vi "步骤循环执行.vi"(0 "通知器输出":refnum<notifier>, 1 "停止":bool, 3 "error in (no error)":errorcluster caption="错误输入（无错误）") -> (7 "组合框":string(combo)="暂停", 10 "error out":errorcluster caption="错误输出")   [LabVIEW 2016]
panel:
  out "报警器":i32
  out "电磁阀2":i32
  out "电磁阀1":i32
  out "蠕动泵":i32
  out "气泵":i32
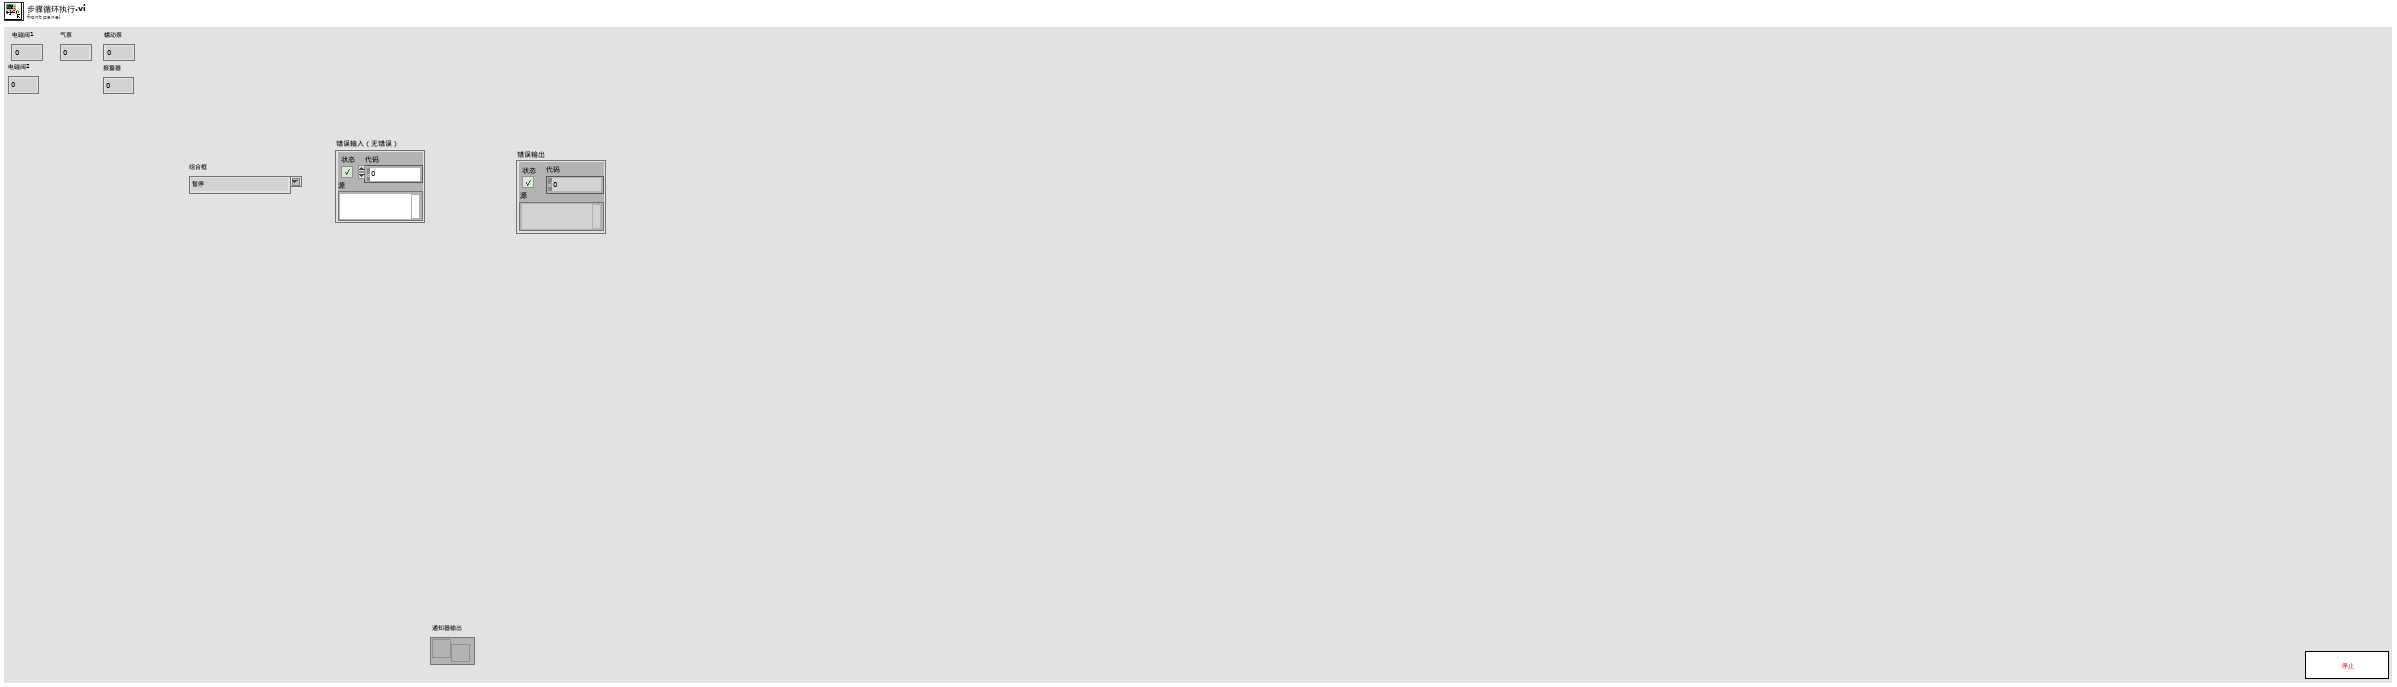
[diagram p1: front panel]
types:
  T1 = enum8{"Enabled", "Disabled", "Disabled and Grayed Out"}
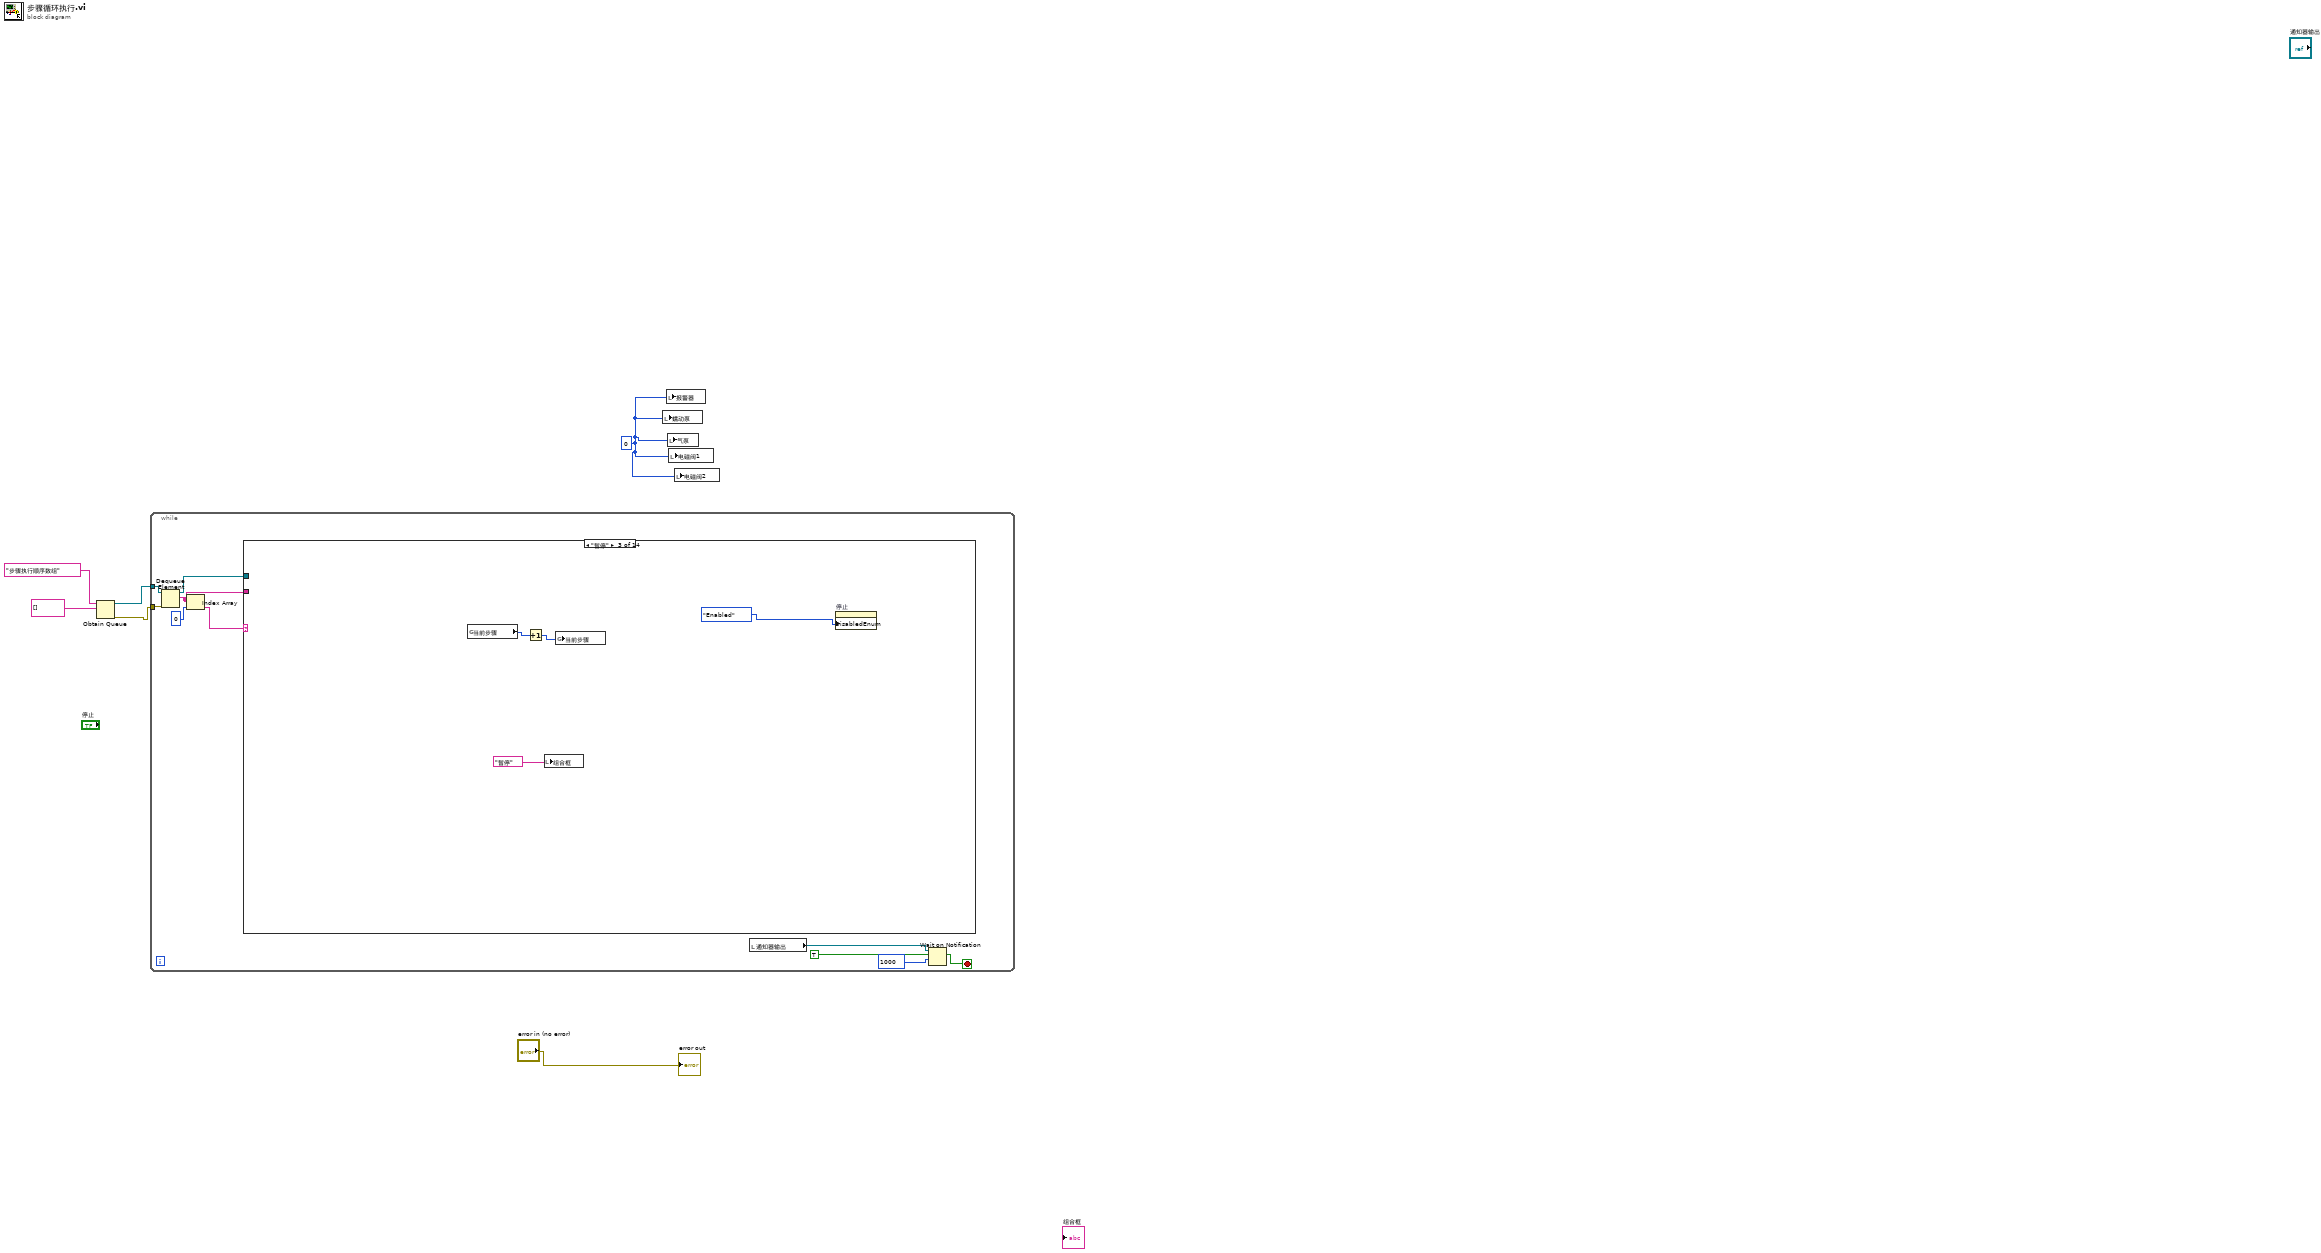
[diagram p0: block diagram]
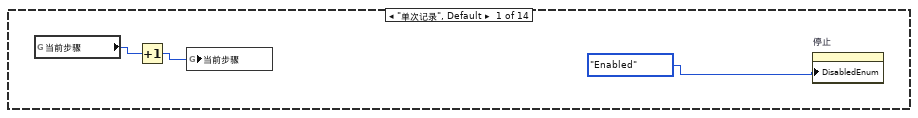
[diagram p2: hidden frame]
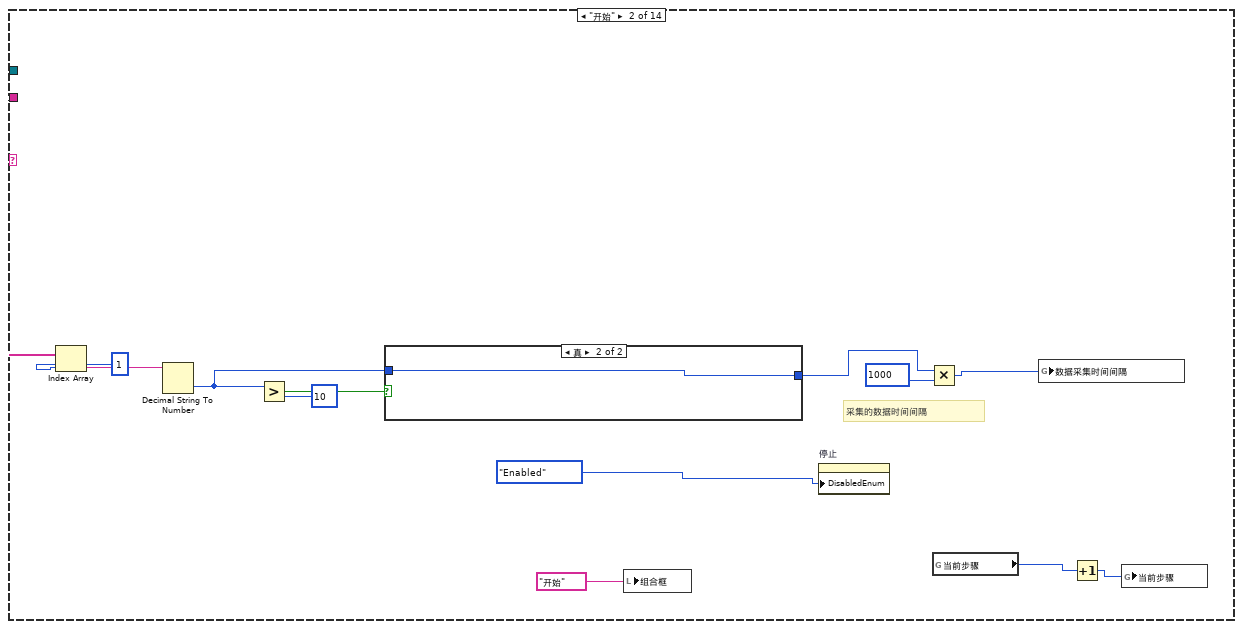
[diagram p3: hidden frame]
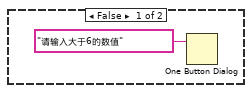
[diagram p4: hidden frame]
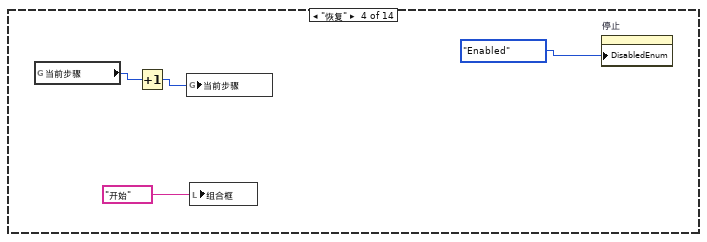
[diagram p5: hidden frame]
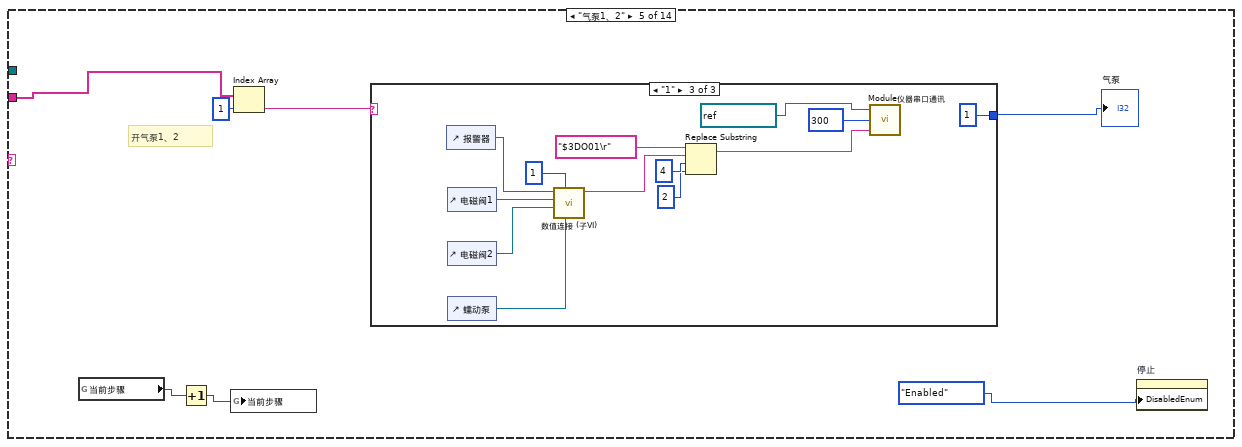
[diagram p6: hidden frame]
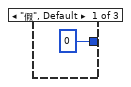
[diagram p7: hidden frame]
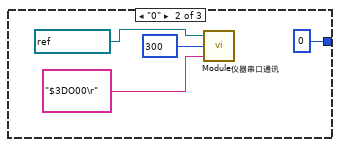
[diagram p8: hidden frame]
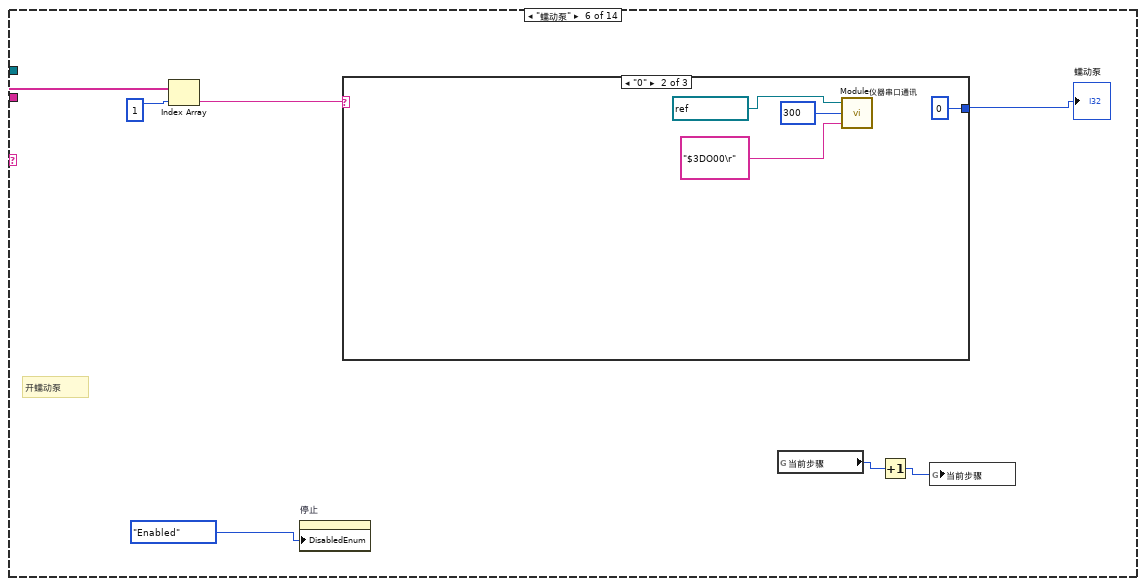
[diagram p9: hidden frame]
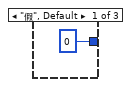
[diagram p10: hidden frame]
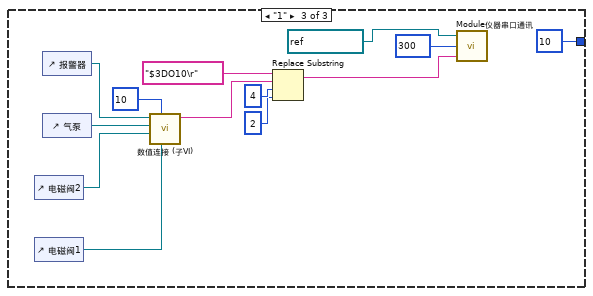
[diagram p11: hidden frame]
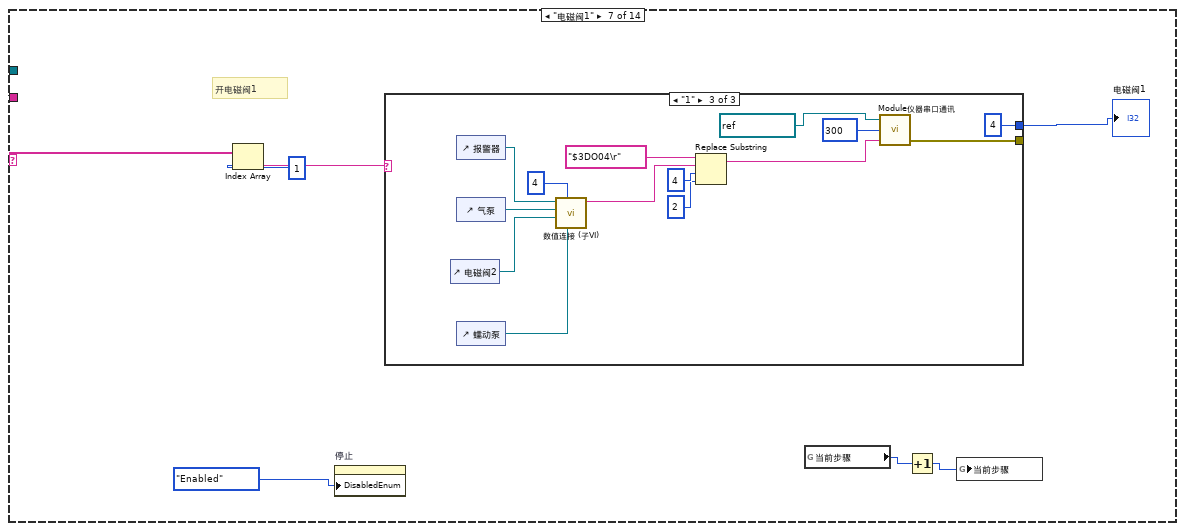
[diagram p12: hidden frame]
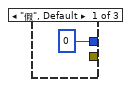
[diagram p13: hidden frame]
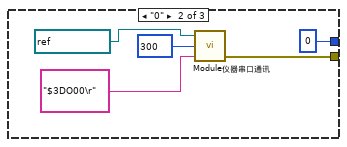
[diagram p14: hidden frame]
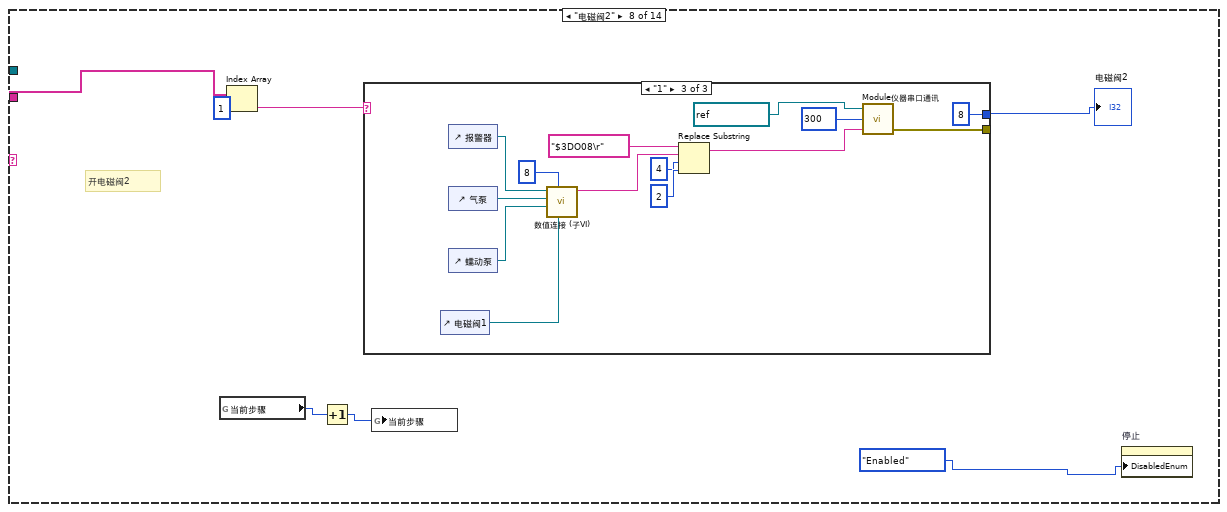
[diagram p15: hidden frame]
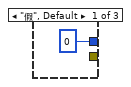
[diagram p16: hidden frame]
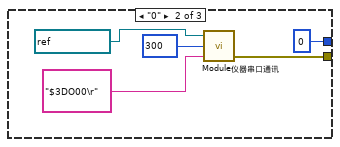
[diagram p17: hidden frame]
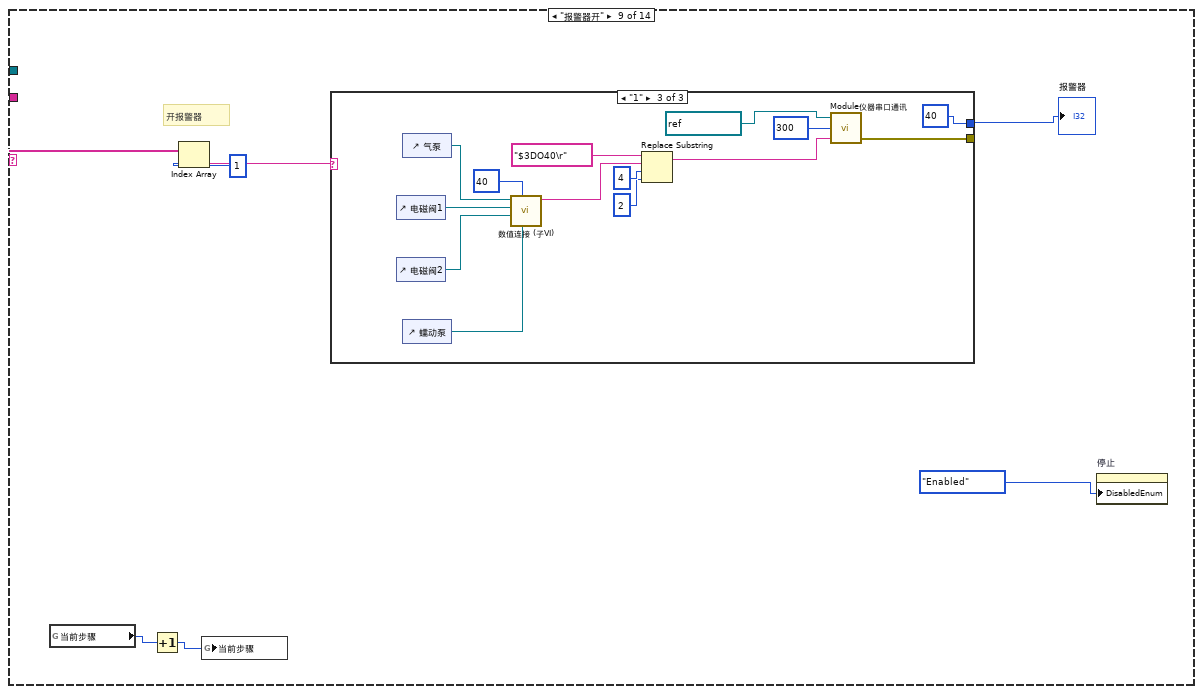
[diagram p18: hidden frame]
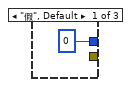
[diagram p19: hidden frame]
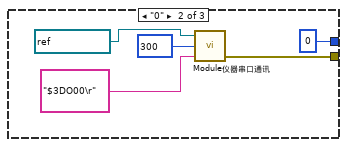
[diagram p20: hidden frame]
diagram:
  w2 = 0
  n1 = Obtain Queue(name (unnamed)="步骤执行顺序数组" ("名称（未命名）"), element data type=string[] [] ("添加的数组 2")) -> (queue out=w5:refnum<queue>, error out=w4:errorcluster)  [unwired: 3 in, 1 out]
  n2 = while {
    tunnel: w5 -> [w16]
    tunnel: w4 -> [w15]
    stop <- w7 stop-if-true
    n3 = Dequeue Element(queue=w16, error in (no error)=w15) -> (queue out=w11:refnum<queue>, element=w12:string[])  [unwired: 1 in, 2 out]
    n4 = Index Array(array=w12, index=0 ("索引")) -> (element=w13:string)
    n5 = case shown="\"暂停\"" w13 {
      tunnel: w12 -> [_ w25 _ _ w49 w71 w96 w123 w150 w177 w191 w221 w235 w246]
      tunnel: w11 -> [_ _ _ _ _ _ _ _ _ _ _ _ w234 _]
      frame "单次记录", Default {
        n6 = global read "全局小变量.vi" "当前步骤"() -> (w19:i32)
        n7 = Increment(x=w19) -> (x+1=w18:i32)
        n8 = global write "全局小变量.vi" "当前步骤"(w18) -> ()
        n9 = property on="停止" class="Bool (严格)"("DisabledEnum"=T1."Enabled" ("禁用")) -> ()  [unwired: 2 in, 2 out]
      }
      frame "开始" {
        # "采集的数据时间间隔"
        n10 = Index Array(array=w25, index=1 ("索引")) -> (element=w27:string)
        n11 = Decimal String To Number(string=w27) -> (number=w32:i32)  [unwired: 2 in, 1 out]
        n12 = Greater?(x=w32, y=10) -> (0:w30:bool)
        n13 = case shown="真" w30 {
          tunnel: [_ w34] -> w31
          tunnel: w32 -> [_ w34]
          frame False {
            n14 = One Button Dialog(message="请输入大于6的数值" ("消息")) -> ()  [unwired: 1 in, 1 out]
          }
          frame True {
          }
        }
        n15 = local write "组合框"("开始" ("组合框")) -> ()
        n16 = property on="停止" class="Bool (严格)"("DisabledEnum"=T1."Enabled" ("禁用")) -> ()  [unwired: 2 in, 2 out]
        n17 = Multiply(x=w31, y=1000) -> (x*y=w23:i32)
        n18 = global read "全局小变量.vi" "当前步骤"() -> (w22:i32)
        n19 = global write "全局小变量.vi" "数据采集时间间隔"(w23) -> ()
        n20 = Increment(x=w22) -> (x+1=w21:i32)
        n21 = global write "全局小变量.vi" "当前步骤"(w21) -> ()
      }
      frame "暂停" {
        n22 = global read "全局小变量.vi" "当前步骤"() -> (w37:i32)
        n23 = Increment(x=w37) -> (x+1=w36:i32)
        n24 = local write "组合框"("暂停" ("组合框")) -> ()
        n25 = global write "全局小变量.vi" "当前步骤"(w36) -> ()
        n26 = property on="停止" class="Bool (严格)"("DisabledEnum"=T1."Enabled" ("禁用")) -> ()  [unwired: 2 in, 2 out]
      }
      frame "恢复" {
        n27 = global read "全局小变量.vi" "当前步骤"() -> (w41:i32)
        n28 = Increment(x=w41) -> (x+1=w40:i32)
        n29 = global write "全局小变量.vi" "当前步骤"(w40) -> ()
        n30 = local write "组合框"("开始" ("组合框")) -> ()
        n31 = property on="停止" class="Bool (严格)"("DisabledEnum"=T1."Enabled" ("禁用")) -> ()  [unwired: 2 in, 2 out]
      }
      frame "气泵1、2" {
        # "开气泵1、2"
        n32 = global read "全局小变量.vi" "当前步骤"() -> (w45:i32)
        n33 = Increment(x=w45) -> (x+1=w44:i32)
        n34 = global write "全局小变量.vi" "当前步骤"(w44) -> ()
        n35 = Index Array(array=w49, index=1 ("索引")) -> (element=w47:string)
        n36 = case shown="\"1\"" w47 {
          tunnel: [0 0 1] -> w46
          frame "假", Default {
          }
          frame "0" {
            n37 = call "Module仪器串口通讯.vi"("输入指令"="$3DO00\r", "baud rate"=u32 300 ("baud rate (9600)"), "VISA resource name"=refnum<visa-resource-name> "COM3") -> ()  [unwired: 3 out]
          }
          frame "1" {
            n38 = control-ref of="报警器"() -> (w58:refnum<vi>)
            n39 = control-ref of="电磁阀1"() -> (w57:refnum<vi>)
            n40 = control-ref of="电磁阀2"() -> (w56:refnum<vi>)
            n41 = control-ref of="蠕动泵"() -> (w55:refnum<vi>)
            n42 = call "数值连接 (子VI).vi"("DigNum引用句柄 4"=w55, "x"=1, "DigNum引用句柄 3"=w56, "DigNum引用句柄输入"=w57, "Digital输入"=w58) -> ("数据字符串"=w61:string)  [unwired: 6 in]
            n43 = Replace Substring(2:2 ("长度（子字符串长度）"), 3:4 ("偏移量(0)"), 4:w61, 5:"$3DO01\r" ("输入指令")) -> (1:w60:string)  [unwired: 1 out]
            n44 = call "Module仪器串口通讯.vi"("输入指令"=w60, "baud rate"=u32 300 ("baud rate (9600)"), "VISA resource name"=refnum<visa-resource-name> "COM3") -> ()  [unwired: 3 out]
          }
        }
        "气泵" <- w46
        n45 = property on="停止" class="Bool (严格)"("DisabledEnum"=T1."Enabled" ("禁用")) -> ()  [unwired: 2 in, 2 out]
      }
      frame "蠕动泵" {
        # "开蠕动泵"
        n46 = Index Array(array=w71, index=1 ("索引")) -> (element=w73:string)
        n47 = property on="停止" class="Bool (严格)"("DisabledEnum"=T1."Enabled" ("禁用")) -> ()  [unwired: 2 in, 2 out]
        n48 = case shown="\"0\"" w73 {
          tunnel: [0 ("电磁阀1") 0 ("电磁阀1") 10 ("电磁阀1")] -> w72
          frame "假", Default {
          }
          frame "0" {
            n49 = call "Module仪器串口通讯.vi"("输入指令"="$3DO00\r", "baud rate"=u32 300 ("baud rate (9600)"), "VISA resource name"=refnum<visa-resource-name> "COM3") -> ()  [unwired: 3 out]
          }
          frame "1" {
            n50 = control-ref of="电磁阀2"() -> (w83:refnum<vi>)
            n51 = control-ref of="电磁阀1"() -> (w80:refnum<vi>)
            n52 = control-ref of="报警器"() -> (w82:refnum<vi>)
            n53 = control-ref of="气泵"() -> (w81:refnum<vi>)
            n54 = call "数值连接 (子VI).vi"("DigNum引用句柄 4"=w80, "x"=10, "DigNum引用句柄 3"=w83, "DigNum引用句柄输入"=w81, "Digital输入"=w82) -> ("数据字符串"=w85:string)  [unwired: 6 in]
            n55 = Replace Substring(2:2 ("长度（子字符串长度）"), 3:4 ("偏移量(0)"), 4:w85, 5:"$3DO10\r" ("输入指令")) -> (1:w87:string)  [unwired: 1 out]
            n56 = call "Module仪器串口通讯.vi"("输入指令"=w87, "baud rate"=u32 300 ("baud rate (9600)"), "VISA resource name"=refnum<visa-resource-name> "COM3") -> ()  [unwired: 3 out]
          }
        }
        "蠕动泵" <- w72
        n57 = global read "全局小变量.vi" "当前步骤"() -> (w70:i32)
        n58 = Increment(x=w70) -> (x+1=w69:i32)
        n59 = global write "全局小变量.vi" "当前步骤"(w69) -> ()
      }
      frame "电磁阀1" {
        # "开电磁阀1"
        n60 = Index Array(array=w96, index=1 ("索引")) -> (element=w98:string)
        n61 = property on="停止" class="Bool (严格)"("DisabledEnum"=T1."Enabled" ("禁用")) -> ()  [unwired: 2 in, 2 out]
        n62 = case shown="\"1\"" w98 {
          tunnel: [_ w102 w117] -> _
          tunnel: [0 0 4 ("电磁阀1")] -> w97
          frame "假", Default {
          }
          frame "0" {
            n63 = call "Module仪器串口通讯.vi"("输入指令"="$3DO00\r", "baud rate"=u32 300 ("baud rate (9600)"), "VISA resource name"=refnum<visa-resource-name> "COM3") -> ("错误输出"=w102:errorcluster)  [unwired: 2 out]
          }
          frame "1" {
            n64 = control-ref of="电磁阀2"() -> (w107:refnum<vi>)
            n65 = control-ref of="报警器"() -> (w109:refnum<vi>)
            n66 = control-ref of="气泵"() -> (w108:refnum<vi>)
            n67 = control-ref of="蠕动泵"() -> (w106:refnum<vi>)
            n68 = call "数值连接 (子VI).vi"("DigNum引用句柄 4"=w106, "x"=4, "DigNum引用句柄 3"=w107, "DigNum引用句柄输入"=w108, "Digital输入"=w109) -> ("数据字符串"=w114:string)  [unwired: 6 in]
            n69 = Replace Substring(2:2 ("长度（子字符串长度）"), 3:4 ("偏移量(0)"), 4:w114, 5:"$3DO04\r" ("输入指令")) -> (1:w111:string)  [unwired: 1 out]
            n70 = call "Module仪器串口通讯.vi"("输入指令"=w111, "baud rate"=u32 300 ("baud rate (9600)"), "VISA resource name"=refnum<visa-resource-name> "COM3") -> ("错误输出"=w117:errorcluster)  [unwired: 2 out]
          }
        }
        "电磁阀1" <- w97
        n71 = global read "全局小变量.vi" "当前步骤"() -> (w95:i32)
        n72 = Increment(x=w95) -> (x+1=w94:i32)
        n73 = global write "全局小变量.vi" "当前步骤"(w94) -> ()
      }
      frame "电磁阀2" {
        # "开电磁阀2"
        n74 = global read "全局小变量.vi" "当前步骤"() -> (w122:i32)
        n75 = Index Array(array=w123, index=1 ("索引")) -> (element=w125:string)
        n76 = Increment(x=w122) -> (x+1=w121:i32)
        n77 = case shown="\"1\"" w125 {
          tunnel: [_ w129 w144] -> _
          tunnel: [0 ("电磁阀1") 0 ("电磁阀1") 8 ("电磁阀1")] -> w124
          frame "假", Default {
          }
          frame "0" {
            n78 = call "Module仪器串口通讯.vi"("输入指令"="$3DO00\r", "baud rate"=u32 300 ("baud rate (9600)"), "VISA resource name"=refnum<visa-resource-name> "COM3") -> ("错误输出"=w129:errorcluster)  [unwired: 2 out]
          }
          frame "1" {
            n79 = control-ref of="电磁阀1"() -> (w135:refnum<vi>)
            n80 = control-ref of="报警器"() -> (w133:refnum<vi>)
            n81 = control-ref of="气泵"() -> (w134:refnum<vi>)
            n82 = control-ref of="蠕动泵"() -> (w136:refnum<vi>)
            n83 = call "数值连接 (子VI).vi"("DigNum引用句柄 4"=w135, "x"=8, "DigNum引用句柄 3"=w136, "DigNum引用句柄输入"=w134, "Digital输入"=w133) -> ("数据字符串"=w141:string)  [unwired: 6 in]
            n84 = Replace Substring(2:2 ("长度（子字符串长度）"), 3:4 ("偏移量(0)"), 4:w141, 5:"$3DO08\r" ("输入指令")) -> (1:w139:string)  [unwired: 1 out]
            n85 = call "Module仪器串口通讯.vi"("输入指令"=w139, "baud rate"=u32 300 ("baud rate (9600)"), "VISA resource name"=refnum<visa-resource-name> "COM3") -> ("错误输出"=w144:errorcluster)  [unwired: 2 out]
          }
        }
        "电磁阀2" <- w124
        n86 = global write "全局小变量.vi" "当前步骤"(w121) -> ()
        n87 = property on="停止" class="Bool (严格)"("DisabledEnum"=T1."Enabled" ("禁用")) -> ()  [unwired: 2 in, 2 out]
      }
      frame "报警器开" {
        # "开报警器"
        n88 = global read "全局小变量.vi" "当前步骤"() -> (w149:i32)
        n89 = Increment(x=w149) -> (x+1=w148:i32)
        n90 = Index Array(array=w150, index=1 ("索引")) -> (element=w152:string)
        n91 = global write "全局小变量.vi" "当前步骤"(w148) -> ()
        n92 = case shown="\"1\"" w152 {
          tunnel: [_ w156 w171] -> _
          tunnel: [0 ("电磁阀1") 0 ("电磁阀1") 40 ("电磁阀1")] -> w151
          frame "假", Default {
          }
          frame "0" {
            n93 = call "Module仪器串口通讯.vi"("输入指令"="$3DO00\r", "baud rate"=u32 300 ("baud rate (9600)"), "VISA resource name"=refnum<visa-resource-name> "COM3") -> ("错误输出"=w156:errorcluster)  [unwired: 2 out]
          }
          frame "1" {
            n94 = control-ref of="电磁阀1"() -> (w162:refnum<vi>)
            n95 = control-ref of="电磁阀2"() -> (w161:refnum<vi>)
            n96 = control-ref of="气泵"() -> (w163:refnum<vi>)
            n97 = control-ref of="蠕动泵"() -> (w160:refnum<vi>)
            n98 = call "数值连接 (子VI).vi"("DigNum引用句柄 4"=w160, "x"=40, "DigNum引用句柄 3"=w161, "DigNum引用句柄输入"=w162, "Digital输入"=w163) -> ("数据字符串"=w169:string)  [unwired: 6 in]
            n99 = Replace Substring(2:2 ("长度（子字符串长度）"), 3:4 ("偏移量(0)"), 4:w169, 5:"$3DO40\r" ("输入指令")) -> (1:w165:string)  [unwired: 1 out]
            n100 = call "Module仪器串口通讯.vi"("输入指令"=w165, "baud rate"=u32 300 ("baud rate (9600)"), "VISA resource name"=refnum<visa-resource-name> "COM3") -> ("错误输出"=w171:errorcluster)  [unwired: 2 out]
          }
        }
        "报警器" <- w151
        n101 = property on="停止" class="Bool (严格)"("DisabledEnum"=T1."Enabled" ("禁用")) -> ()  [unwired: 2 in, 2 out]
      }
      frame "报警器关" {
        # "关报警器"
        n102 = global read "全局小变量.vi" "当前步骤"() -> (w176:i32)
        n103 = Index Array(array=w177, index=1 ("索引")) -> (element=w178:string)
        n104 = Increment(x=w176) -> (x+1=w175:i32)
        n105 = global write "全局小变量.vi" "当前步骤"(w175) -> ()
        n106 = case shown="\"0\"" w178 {
          tunnel: [_ w180 w184] -> _
          frame "假", Default {
          }
          frame "0" {
            n107 = call "Module仪器串口通讯.vi"("输入指令"="$3DO00\r", "baud rate"=u32 300 ("baud rate (9600)"), "VISA resource name"=refnum<visa-resource-name> "COM3") -> ("错误输出"=w180:errorcluster)  [unwired: 2 out]
          }
          frame "1" {
            n108 = call "Module仪器串口通讯.vi"("输入指令"="$3DO80\r", "baud rate"=u32 300 ("baud rate (9600)"), "VISA resource name"=refnum<visa-resource-name> "COM3") -> ("错误输出"=w184:errorcluster)  [unwired: 2 out]
          }
        }
        n109 = property on="停止" class="Bool (严格)"("DisabledEnum"=T1."Enabled" ("禁用")) -> ()  [unwired: 2 in, 2 out]
      }
      frame "Set Valve Position" {
        n110 = Index Array(array=w191, index=1 ("索引")) -> (element=w192:string)
        n111 = Equal?(x=w192, y="1") -> (x = y?=w199:bool)
        n112 = Equal?(x=w192, y="3") -> (x = y?=w198:bool)
        n113 = Equal?(x=w192, y="5") -> (x = y?=w196:bool)
        n114 = Equal?(x=w192, y="7") -> (x = y?=w194:bool)
        n115 = case shown="真" w199 {
          tunnel: [_ w215] -> _
          tunnel: w192 -> [_ w214]
          frame False {
          }
          frame True {
            n116 = global write "全局小变量.vi" "多位阀的位置"(w214) -> ()
            n117 = call "VICI仪器串口通讯.vi"("输入指令"="CW1\n\r", "VISA resource name"=refnum<visa-resource-name> "COM1") -> ("错误输出"=w215:errorcluster)  [unwired: 1 in, 2 out]
          }
        }
        n118 = case shown="真" w198 {
          tunnel: [_ w211] -> _
          tunnel: w192 -> [_ w210]
          frame False {
          }
          frame True {
            n119 = global write "全局小变量.vi" "多位阀的位置"(w210) -> ()
            n120 = call "VICI仪器串口通讯.vi"("输入指令"="CW3\n\r", "VISA resource name"=refnum<visa-resource-name> "COM1") -> ("错误输出"=w211:errorcluster)  [unwired: 1 in, 2 out]
          }
        }
        n121 = case shown="真" w196 {
          tunnel: [_ w207] -> _
          tunnel: w192 -> [_ w206]
          frame False {
          }
          frame True {
            n122 = global write "全局小变量.vi" "多位阀的位置"(w206) -> ()
            n123 = call "VICI仪器串口通讯.vi"("输入指令"="CW5\n\r", "VISA resource name"=refnum<visa-resource-name> "COM1") -> ("错误输出"=w207:errorcluster)  [unwired: 1 in, 2 out]
          }
        }
        n124 = case shown="真" w194 {
          tunnel: [_ w203] -> _
          tunnel: w192 -> [_ w202]
          frame False {
          }
          frame True {
            n125 = global write "全局小变量.vi" "多位阀的位置"(w202) -> ()
            n126 = call "VICI仪器串口通讯.vi"("输入指令"="CW7\n\r", "VISA resource name"=refnum<visa-resource-name> "COM1") -> ("错误输出"=w203:errorcluster)  [unwired: 1 in, 2 out]
          }
        }
        n127 = global read "全局小变量.vi" "当前步骤"() -> (w190:i32)
        n128 = Increment(x=w190) -> (x+1=w189:i32)
        n129 = global write "全局小变量.vi" "当前步骤"(w189) -> ()
        n130 = property on="停止" class="Bool (严格)"("DisabledEnum"=T1."Enabled" ("禁用")) -> ()  [unwired: 2 in, 2 out]
      }
      frame "Read All sensor Values" {
        n131 = Index Array(array=w221, index=1 ("索引")) -> (element=w224:string)
        n132 = global read "全局小变量.vi" "当前步骤"() -> (w220:i32)
        n133 = Equal?(x=w224, y="1") -> (x = y?=w222:bool)
        n134 = case shown="假" w222 {
          frame False {
            w226 = "" ("T(cool)℃")
            n135 = global write "全局小变量.vi" "F(Flow)ml/min"(w226) -> ()
            n136 = global write "全局小变量.vi" "P（eq)mv"(w226) -> ()
            n137 = global write "全局小变量.vi" "R(Gas)mv"(w226) -> ()
            n138 = global write "全局小变量.vi" "T(cool)℃"(w226) -> ()
          }
          frame True {
            # "读取流量传感器"
            n139 = call "读取流量传感器(子VI).vi"() -> ("R(Gas)mv"=w229:string, "F(Flow)ml/min"=w228:string, "P（eq)mv"=w227:string, "T(cool)℃"=w230:string)  [unwired: 7 in, 1 out]
            n140 = global write "全局小变量.vi" "F(Flow)ml/min"(w228) -> ()
            n141 = global write "全局小变量.vi" "T(cool)℃"(w230) -> ()
            n142 = global write "全局小变量.vi" "P（eq)mv"(w227) -> ()
            n143 = global write "全局小变量.vi" "R(Gas)mv"(w229) -> ()
          }
        }
        n144 = Increment(x=w220) -> (x+1=w219:i32)
        n145 = global write "全局小变量.vi" "当前步骤"(w219) -> ()
        n146 = property on="停止" class="Bool (严格)"("DisabledEnum"=T1."Enabled" ("禁用")) -> ()  [unwired: 2 in, 2 out]
      }
      frame "等待" {
        n147 = flat-sequence {
          tunnel: w235 -> [w236]
          tunnel: w234 -> [w242]
          frame #0 {
            n148 = Index Array(array=w236, index=1 ("索引")) -> (element=w240:string)
            n149 = Decimal String To Number(string=w240) -> (number=w239:i32)  [unwired: 2 in, 1 out]
            n150 = Multiply(x=w239, y=60000) -> (x*y=w237:i32)
            n151 = Wait (ms)(milliseconds to wait=w237) -> ()  [unwired: 1 out]
          }
          frame #1 {
            n152 = Flush Queue(queue=w242) -> ()  [unwired: 1 in, 3 out]
          }
        }
        n153 = global read "全局小变量.vi" "当前步骤"() -> (w233:i32)
        n154 = Increment(x=w233) -> (x+1=w232:i32)
        n155 = global write "全局小变量.vi" "当前步骤"(w232) -> ()
        n156 = property on="停止" class="Bool (严格)"("DisabledEnum"=T1."Disabled and Grayed Out" ("禁用")) -> ()  [unwired: 2 in, 2 out]
      }
      frame "跳转事件" {
        # "跳转次数"
        n157 = Index Array(array=w246, index=2 ("索引")) -> (element=w247:string)
        n158 = Decimal String To Number(string=w247) -> (number=w245:i32)  [unwired: 2 in, 1 out]
        n159 = Equal To 0?(x=w245) -> (x = 0?=w244:bool)
        n160 = case shown="假" w244 {
          tunnel: w246 -> [w252 w266]
          tunnel: w245 -> [w251 _]
          frame False {
            n161 = global read "全局小变量.vi" "跳转次数变量"() -> (w250:i32)
            n162 = Greater Or Equal?(x=w250, y=w251) -> (x >= y?=w253:bool)
            n163 = case shown="真" w253 {
              tunnel: w252 -> [w255 _]
              frame False {
                # "跳转"
                n164 = Index Array(array=w255, index=1 ("索引")) -> (element=w257:string)
                n165 = Decimal String To Number(string=w257) -> (number=w254:i32)  [unwired: 2 in, 1 out]
                n166 = global write "全局小变量.vi" "当前步骤"(w254) -> ()
              }
              frame True {
                n167 = global read "全局小变量.vi" "数组大小"() -> (w258:i32)
                n168 = global read "全局小变量.vi" "当前步骤"() -> (w259:i32)
                n169 = Greater Or Equal?(x=w259, y=w258) -> (x >= y?=w260:bool)
                n170 = case shown="假" w260 {
                  frame False {
                    n171 = global read "全局小变量.vi" "当前步骤"() -> (w262:i32)
                    n172 = Increment(x=w262) -> (x+1=w261:i32)
                    n173 = global write "全局小变量.vi" "当前步骤"(w261) -> ()
                  }
                  frame True {
                    n174 = local read "通知器输出"() -> (w263:refnum<notifier>)
                    n175 = Send Notification(notification=TRUE ("通知"), notifier=w263) -> ()  [unwired: 1 in, 2 out]
                  }
                }
              }
            }
            n176 = Increment(x=w250) -> (x+1=w249:i32)
            n177 = global write "全局小变量.vi" "跳转次数变量"(w249) -> ()
          }
          frame True {
            # "跳转"
            n178 = Index Array(array=w266, index=1 ("索引")) -> (element=w268:string)
            n179 = Decimal String To Number(string=w268) -> (number=w265:i32)  [unwired: 2 in, 1 out]
            n180 = global write "全局小变量.vi" "当前步骤"(w265) -> ()
          }
        }
        n181 = property on="停止" class="Bool (严格)"("DisabledEnum"=T1."Enabled" ("禁用")) -> ()  [unwired: 2 in, 2 out]
      }
    }
    n182 = local read "通知器输出"() -> (w10:refnum<notifier>)
    n183 = Wait on Notification(notifier=w10, ignore previous (F)=TRUE, timeout in ms (-1)=u32 1000 ("等待时间（毫秒）")) -> (notification=w7:bool)  [unwired: 1 in, 3 out]
  }
  n184 = local write "蠕动泵"(w2) -> ()
  n185 = local write "报警器"(w2) -> ()
  n186 = local write "气泵"(w2) -> ()
  n187 = local write "电磁阀1"(w2) -> ()
  n188 = local write "电磁阀2"(w2) -> ()
  "error out" <- "error in (no error)"
